vi "set_output.vi"(8 "error in (no error)":errorcluster, 10 "output":i32, 11 "output_request_poller in":refnum<class "output_poller.lvclass">) -> (0 "error out":errorcluster, 3 "output_request_poller out":refnum<class "output_poller.lvclass">)   [LabVIEW 2015, in "output_poller.lvclass"]
uses:
  output_poller.lvclass
  output_poller.lvclass/output_poller.ctl
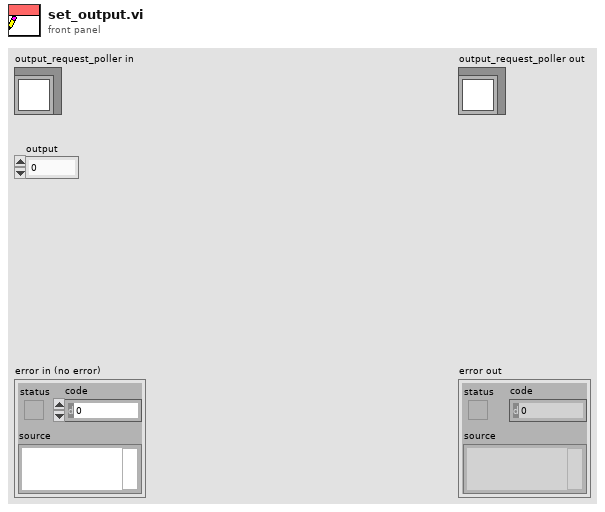
[diagram p1: front panel]
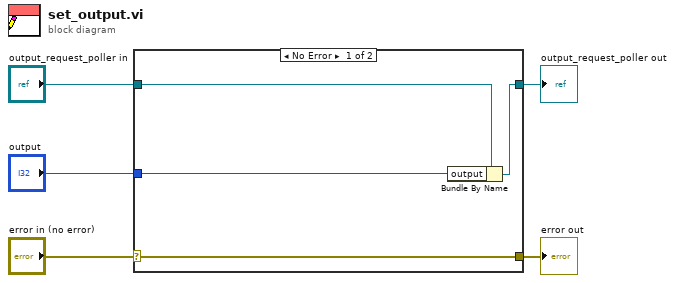
[diagram p0: block diagram]
diagram:
  n1 = case shown="No Error" "error in (no error)" {
    selector: "error in (no error)" -> [w9 w10]
    tunnel: [w9 w10] -> w4
    tunnel: [w7 w11] -> w2
    tunnel: "output_request_poller in" -> [w8 w11]
    tunnel: "output" -> [w6 _]
    frame No Error {
      n2 = Bundle By Name(cluster=w8, "output"=w6) -> (w7:refnum<class "output_poller.lvclass">)
    }
    frame Error {
    }
  }
  "error out" <- w4
  "output_request_poller out" <- w2
